vi "S-TI-S JJ Simulation.vi"() -> ()   [LabVIEW 2023]
doc: "1. before run, set the paramaters on the left of the screen.\n2. flux (magnetic field) is in unit of flux quanta.\n3. Phaserange is in the unit of Pi, the CPR will be build up according to phase range of [-Phaserange/2,Phaserang/2], and such CPR will be a periodic function with Phaserange as period. Enter integer number of multiple times of 4 is preferred.\n4. Use the step setting tab to set resolution of the calculation, you can set how many points is used to define the width of the Josephson junction, how many points to represent the Phaserange\n5. Then you can choose which type of the CPR is used.\n6. Depending on the choose of the CPR, you may want to set the strength of the MBS, \"a\" parameter, the width of the gaussian function used, and the pattern of parity of MBS. Parity pattern has to have same number of elements for positive and negative range.\nEnter the parity 1 or -1 for positive and negative phase +-Pi, +-3Pi, +-5Pi etc.. in to the two arrays.\n7. You can use the index control to read the array elements, then enter the value, you can also delete an element of array by right click, the number of array elements is not limited.\n8. You can change the x,y range, zoom, create cursor etc. to help analyse the plot. Right click to save the data into excel.\n\nEnjoy!\nGuang Yue\ngyue@illinois.edu"
uses:
  dllparameter.ctl
  remove last element_plots.vi
  remove last element_2Darray.vi
panel:
  out "Current Disorder":T1={"Step width"=0.2, "App"=0.1, "Array"=[1.0078411649904462, 1.0078411649904462, 0.9846991573254764, 0.9846991573254764, 0.9978814600222632, 0.9978814600222632, 0.9723089162683902, 0.9723089162683902, 1.011631648566163, 1.011631648566163]}
  in  "Tab Control":T2(tab)
  in  "flux start":dbl=-5.0
  in  "flux end":dbl=5.0
  in  "flux step":dbl=0.1
  in  "Geometry steps":i32=201
  in  "Phase steps":i32=201
  in  "CPR Type":T3(ring)
  in  "CPR plot points":i32=500
  in  "parity for negative phase":i32[](array[numeric])=[1, -1, -1, 1]
  in  "Strenth of MBS":dbl=0.5
  in  "parity for positive phase":i32[](array[numeric])=[1, -1, 1, 1]
  in  "Gaussian width":dbl=0.2
  in  "Plot CPR":bool
  in  "Set Disorder":bool
  out "Actual flux":dbl
  in  "Flux":dbl
  in  "Plot choice":enum32{"Icp", "Icn"}(radio)
  in  "Geometry Disorder Type":u16(ring) items=["Disorder OFF", "Disorder ON"]
  in  "Plot J vs y":bool
  out "error out":errorcluster
  in  "clear last":bool
  in  "clear tab":bool
  in  "clear All":bool
  out "Negative Phase0":dbl
  out "phaserange in Pi":i32=16
  out "Positive Phase0":dbl
  in  "Plot tab":T4(tab)
  out "Diffraction pattern plot":cluster{cluster{dbl, "icn":dbl}[]}[](graph)
  out "Phase0 vs Flux":cluster{cluster{dbl, "icn":dbl}[]}[](graph)
  out "J vs y":cluster{cluster{dbl, "icn":dbl}[]}[](graph)
  out "CPR":cluster{cluster{dbl, "icn":dbl}[]}[](graph)
  out "Disorder":dbl[][](graph)
  in  "Save":bool
  in  "hold":bool=TRUE
  out "Current Flux":dbl=5.0
  out "Remaining steps":i32
  in  "Exit":bool
  in  "Run":bool
  out "Total time s":dbl=5.020437899999706 format="%#_5g"
  in  "stop":bool
  out "Ic negative":dbl=-0.0009989221220817583
  out "Ic positive":dbl=0.000998922122081775 format="%#_5f"
  # "Go to Help menu for instructions, \nor move your mouse cursor on the \nobject for some tip."
  # "Calculate Diffraction pattern"
  # "Version 2.1"
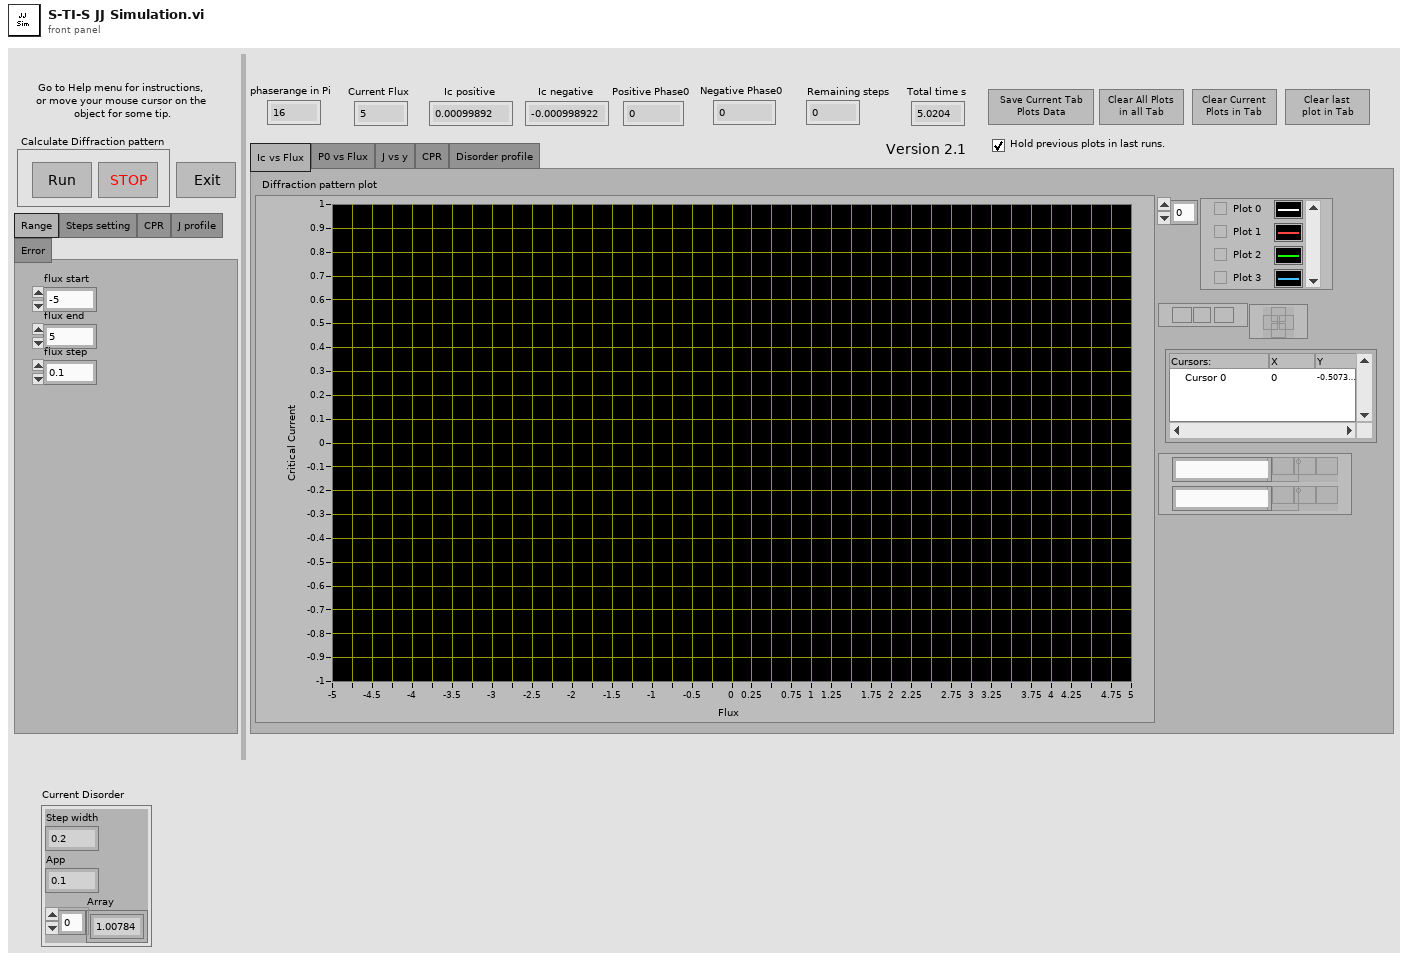
[diagram p1: front panel]
types:
  T1 = cluster{"Step width":dbl, "App":dbl, "Array":dbl[]}
  T2 = enum32{"Range", "Steps setting", "CPR", "J profile", "Error"}
  T3 = enum16{"Regular Josephson effect", "Non-local MBS", "Local MBS same parity", "Local MBS different parity"}
  T4 = enum32{"Ic vs Flux", "P0 vs Flux", "J vs y", "CPR", "Disorder profile"}
  T5 = enum8{"Enabled", "Disabled", "Disabled and Grayed Out"}
  T6 = typedef "dllparameter.ctl" = cluster{"Gaussian width":dbl, "Strenth of MBS":dbl, "Phase steps":i32, "Geometry steps":i32, "Geometry Noise Type":u16, "CPR Type":dbl, "parity for positive phase":dbl[], "parity for negative phase ":dbl[]}
  T7 = cluster{cluster{"phase":dbl, "return type":dbl}[]}
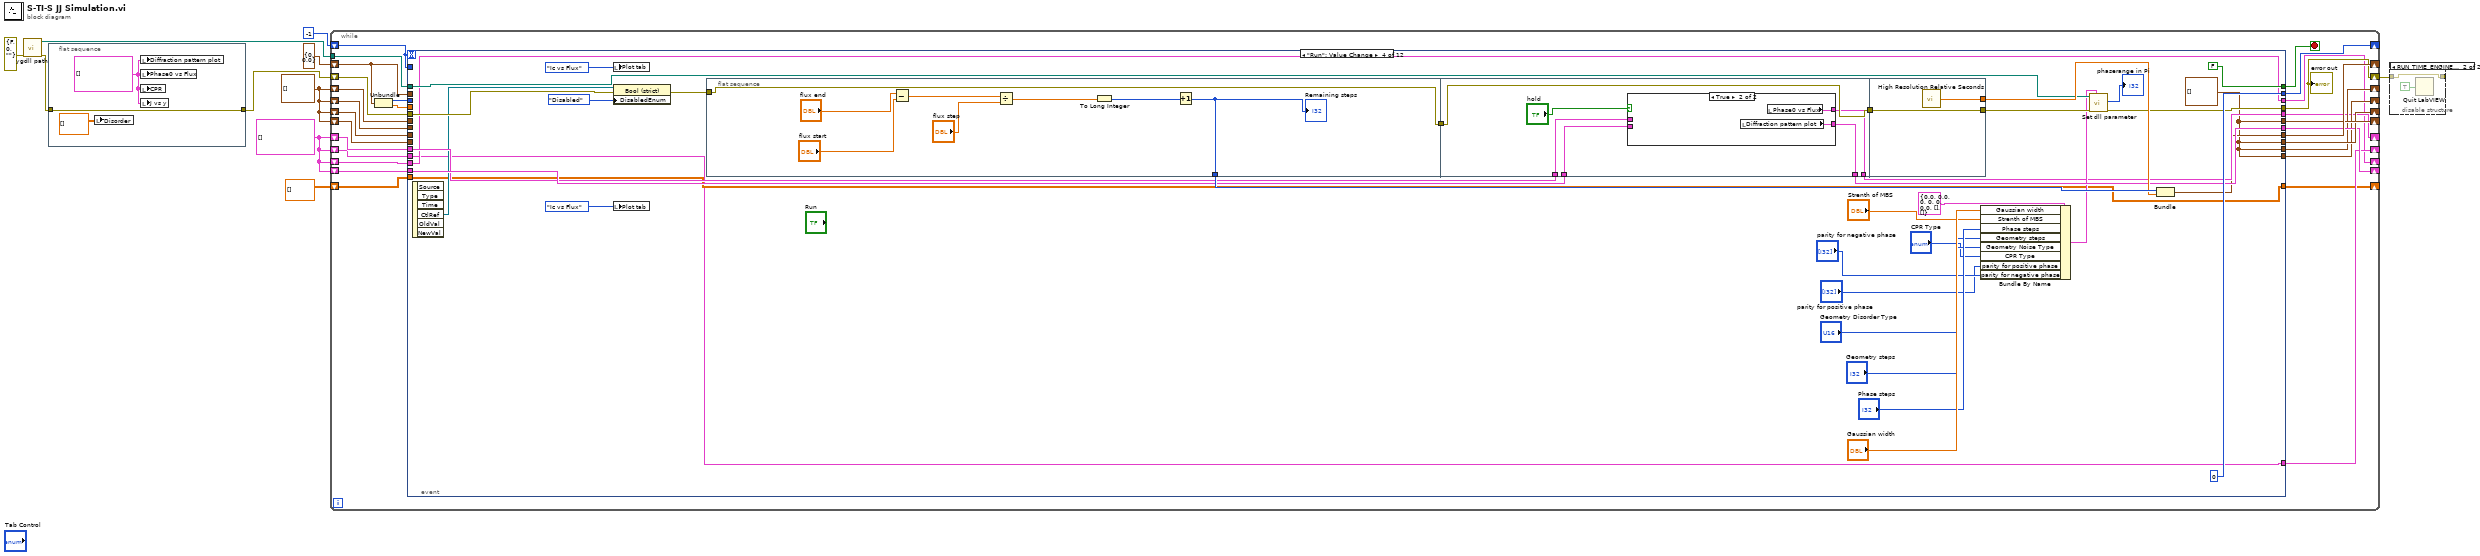
[diagram p0: block diagram]
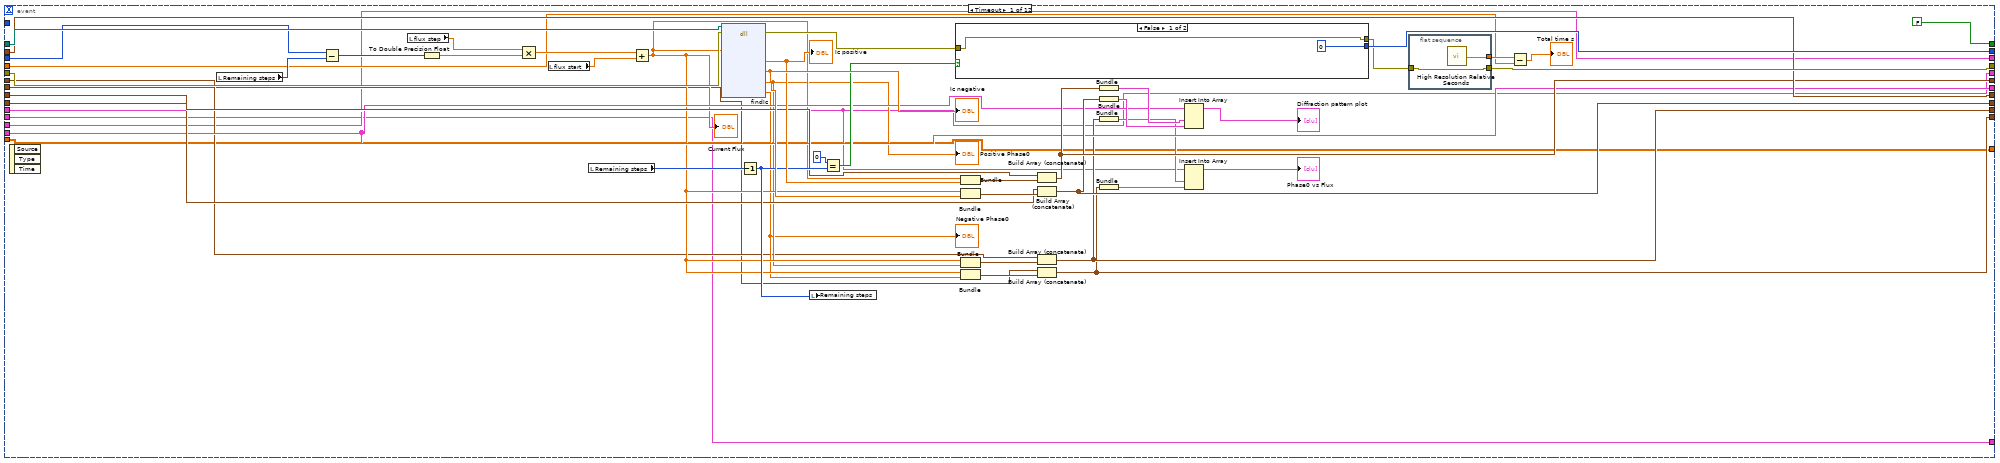
[diagram p3: hidden frame]
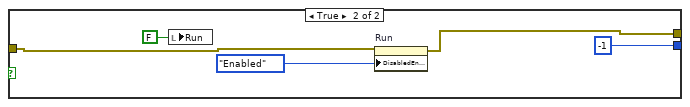
[diagram p4: hidden frame]
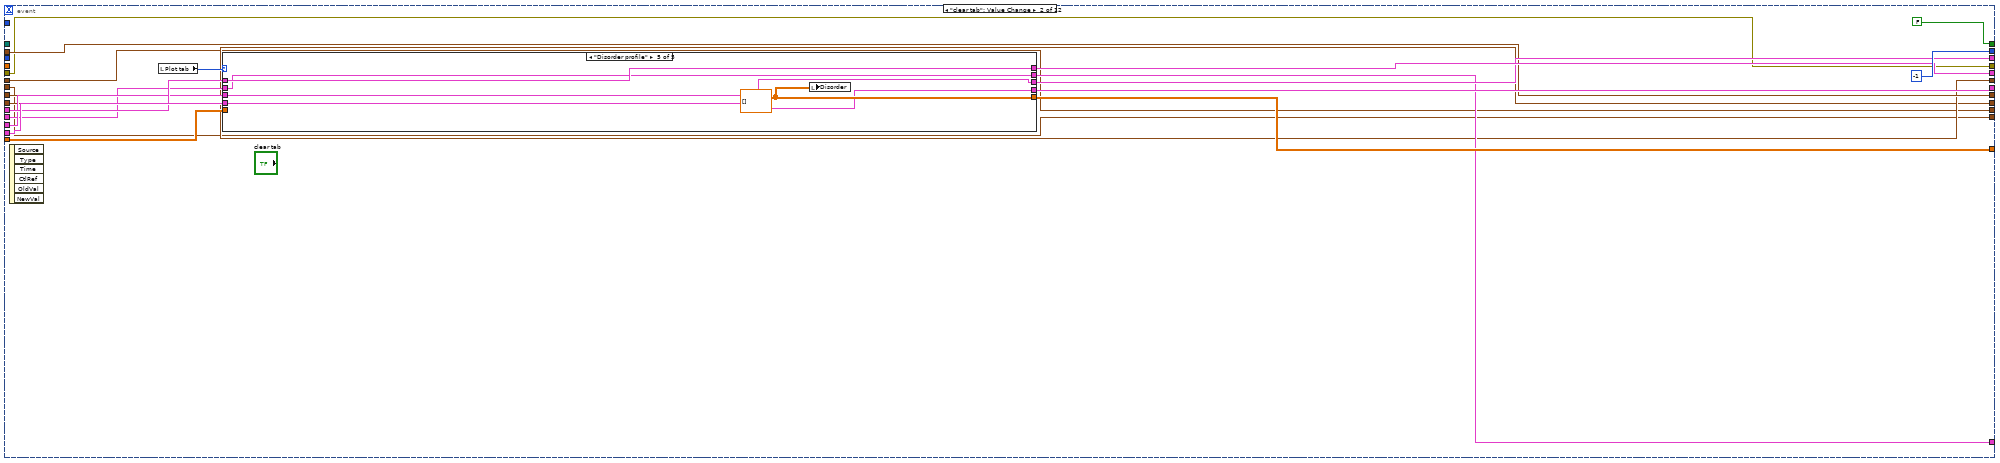
[diagram p5: hidden frame]
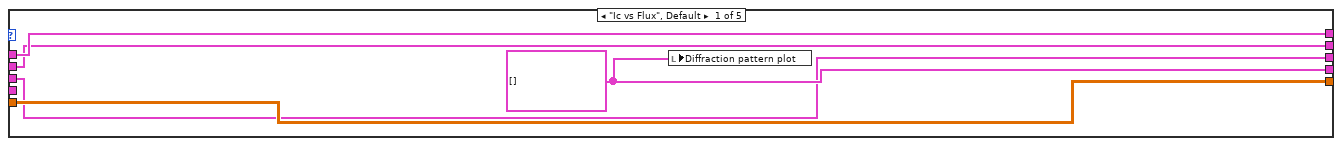
[diagram p6: hidden frame]
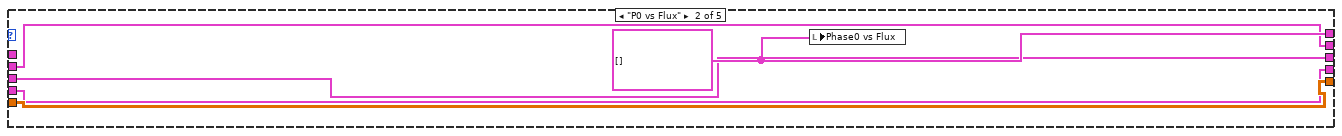
[diagram p7: hidden frame]
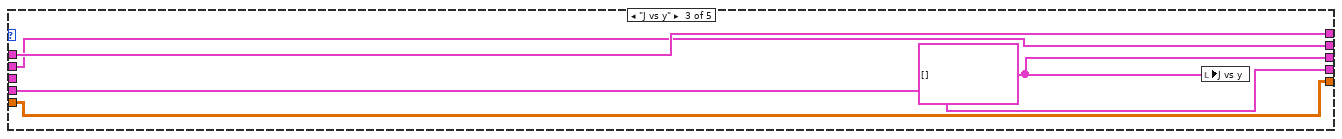
[diagram p8: hidden frame]
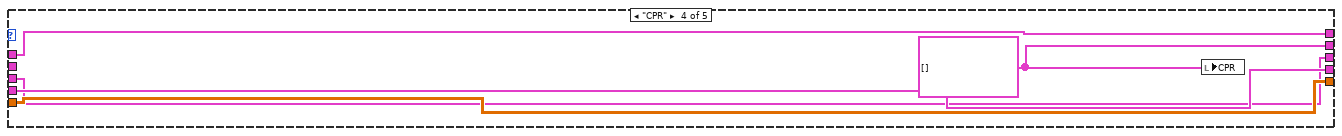
[diagram p9: hidden frame]
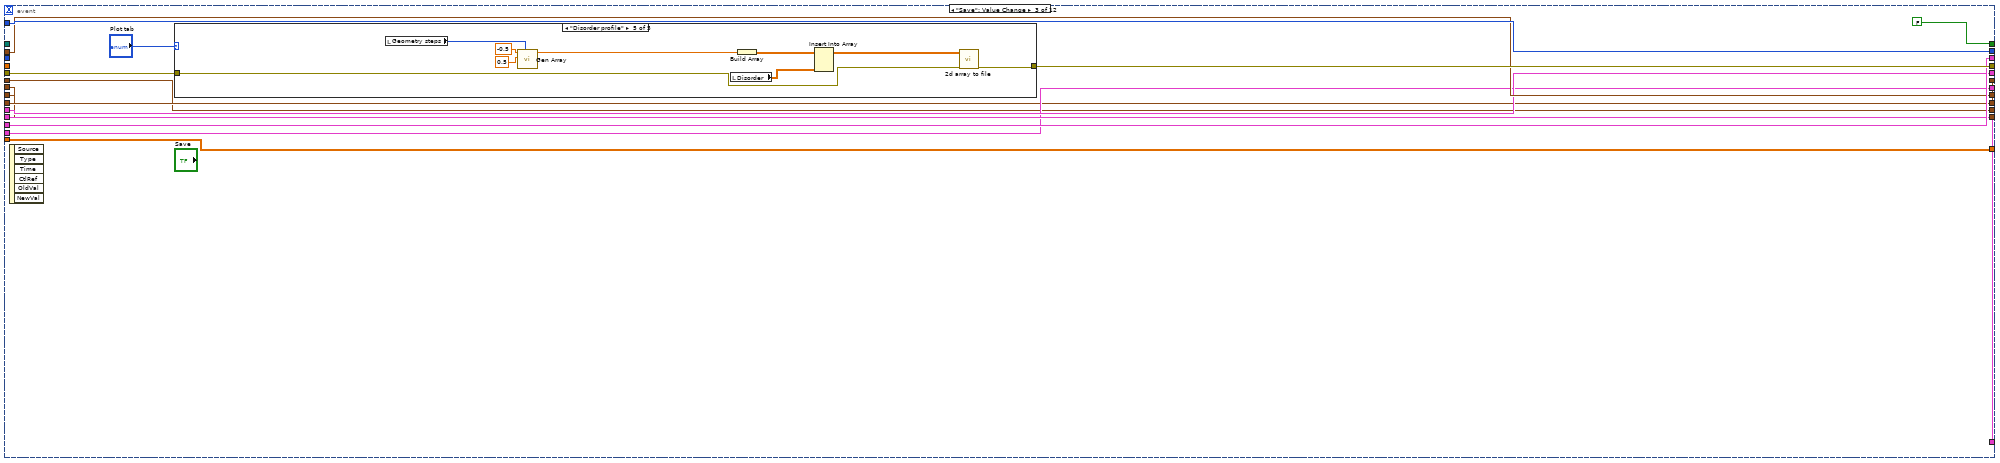
[diagram p10: hidden frame]
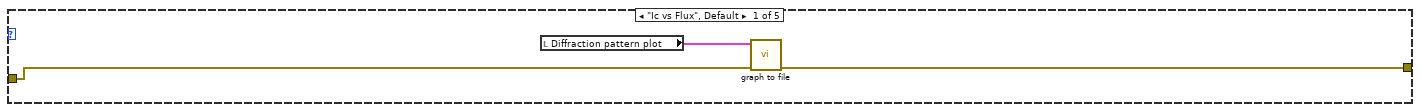
[diagram p11: hidden frame]
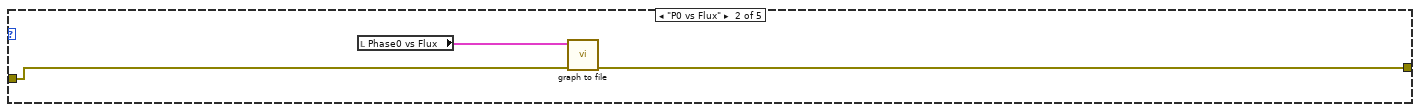
[diagram p12: hidden frame]
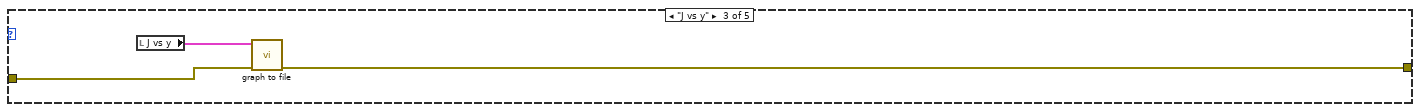
[diagram p13: hidden frame]
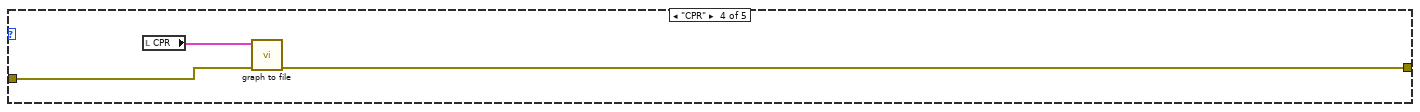
[diagram p14: hidden frame]
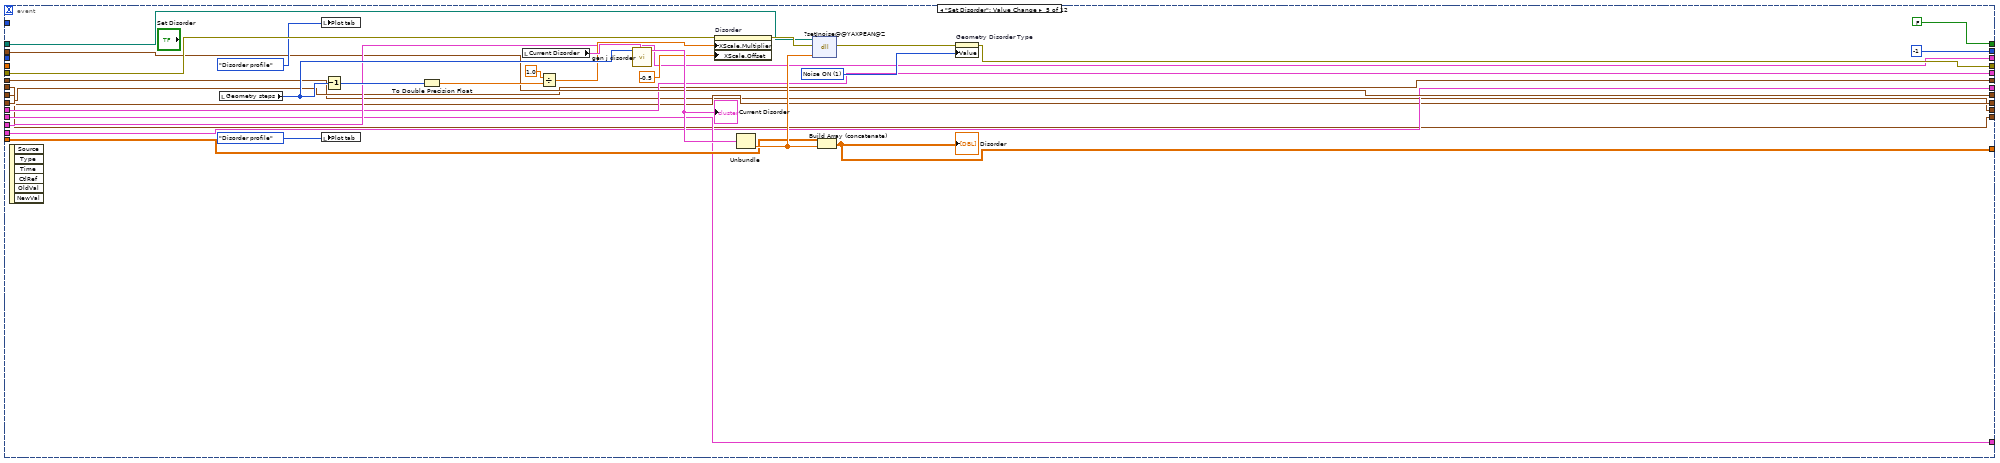
[diagram p16: hidden frame]
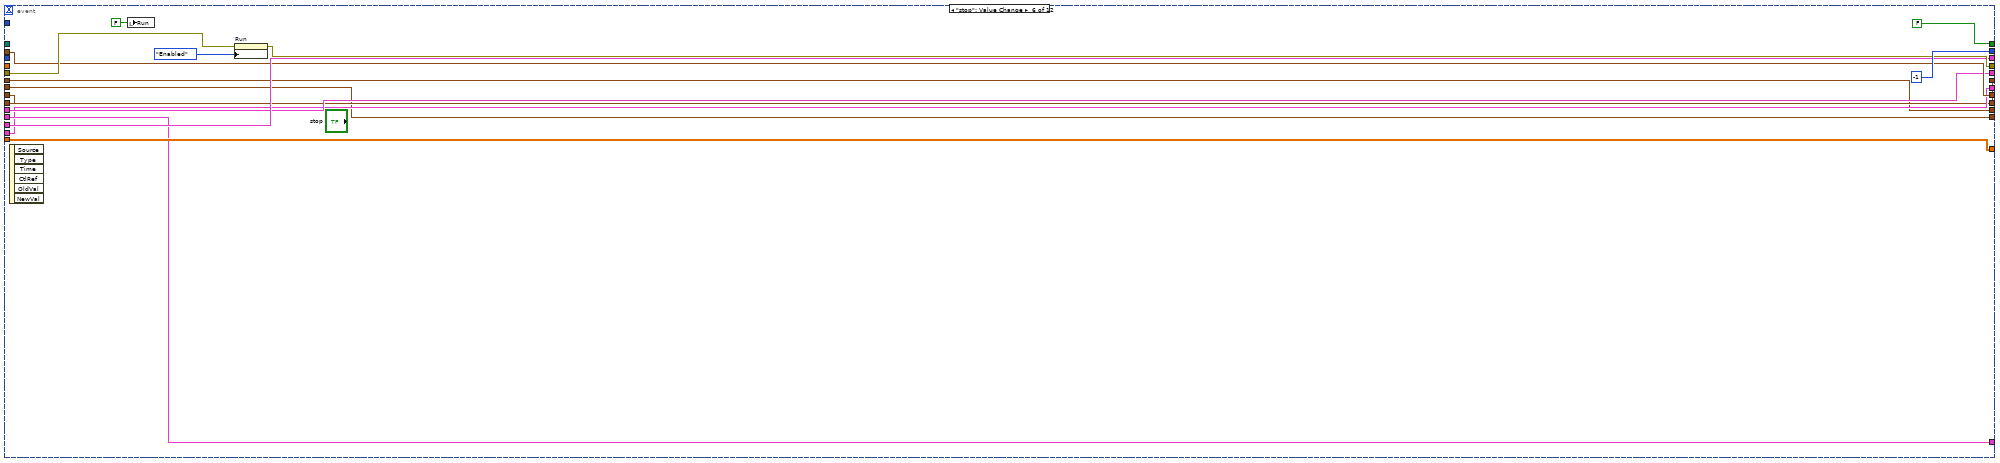
[diagram p17: hidden frame]
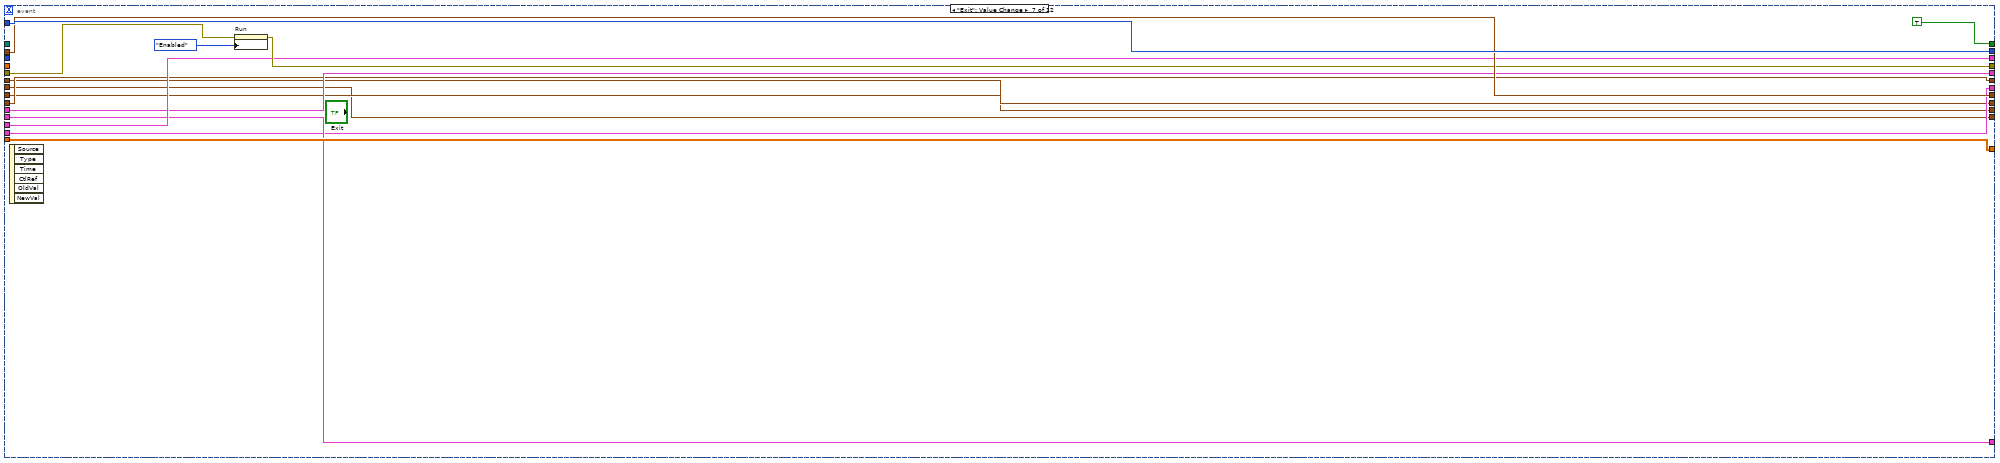
[diagram p18: hidden frame]
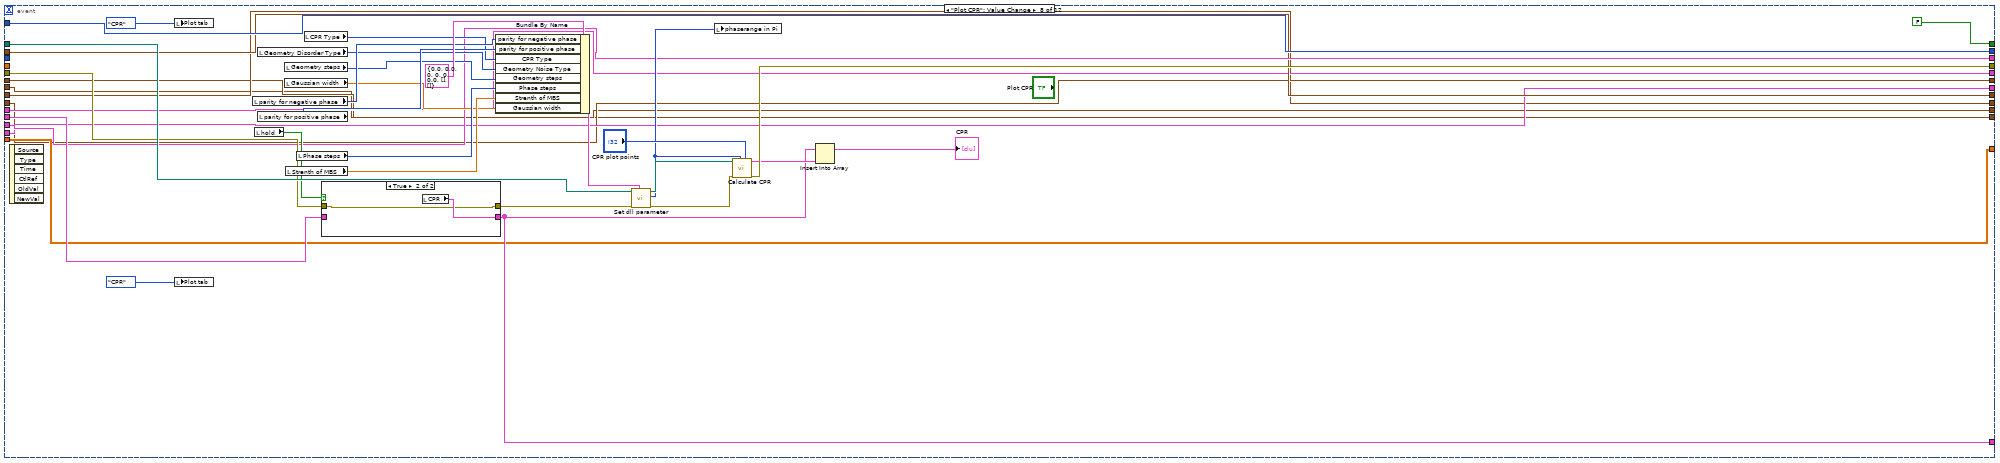
[diagram p19: hidden frame]
diagram:
  w2 = cluster{cluster{dbl, "icn":dbl}[]}[] [] ("appended array")
  w3 = cluster{dbl, "inp":dbl}[] []
  n1 = call "ygdll path.vi"("error in (no error)"=errorcluster {"status"=FALSE, "code"=0, "source"=""} ("error out")) -> ("error out"=w6:errorcluster, "appended path"=w9:path)  [unwired: 9 in]
  n2 = flat-sequence {
    tunnel: w6 -> [w13]
    tunnel: [w13] -> w5
    frame #0 {
      w12 = cluster{cluster{dbl, "icn":dbl}[]}[] [] ("appended array")
      n3 = local write "Disorder"(dbl[][] [] ("Disorder")) -> ()
      n4 = local write "Diffraction pattern plot"(w12) -> ()
      n5 = local write "Phase0 vs Flux"(w12) -> ()
      n6 = local write "CPR"(w12) -> ()
      n7 = local write "J vs y"(w12) -> ()
    }
  }
  n8 = while {
    tunnel: w9 -> [w38]
    shift-right: [w40] -> _
    shift-left: -1 -> [w33]
    shift-right: [w41] -> _
    shift-left: cluster{i32, "relative seconds":dbl} {0, "relative seconds"=0.0} ("output cluster") -> [w34]
    shift-right: [w36] -> w7
    shift-left: w5 -> [w39]
    shift-right: [w31] -> _
    shift-left: w3 -> [w32]
    shift-right: [w30] -> _
    shift-left: w3 -> [w29]
    shift-right: [w26] -> _
    shift-left: w2 -> [w27]
    shift-right: [w23] -> _
    shift-left: w3 -> [w25]
    shift-right: [w22] -> _
    shift-left: w3 -> [w24]
    shift-right: [w20] -> _
    shift-left: w2 -> [w21]
    shift-right: [w18] -> _
    shift-left: w2 -> [w19]
    shift-right: [w16] -> _
    shift-left: w2 -> [w17]
    shift-right: [w14] -> _
    shift-left: dbl[][] [] -> [w15]
    stop <- w28 stop-if-true
    n9 = Unbundle(w34) -> (w35:i32, "relative seconds"=w37:dbl)
    n10 = event shown="[3] \"Run\": Value Change" {
      selector: _ -> [_ _ _ _ _ _ _ _ _ _ _ _]
      dyn-events: _ -> [_ _ _ _ _ _ _ _ _ _ _ _]
      timeout: w33 -> [_ _ _ _ _ _ _ _ _ _ _ _]
      tunnel: [w69 w106 w152 w190 w244 w273 w295 w303 w342 w352 w403 w440] -> w41
      tunnel: [w71 -1 w158 0 -1 -1 w296 w330 -1 -1 -1 w447] -> w40
      tunnel: w39 -> [w84 w105 w156 w211 w255 w280 w293 w313 w341 w351 w411 w446]
      tunnel: w38 -> [w83 _ _ w203 w236 _ _ w328 _ _ w424 _]
      tunnel: w37 -> [w58 _ _ _ _ _ _ _ _ _ _ _]
      tunnel: [w82 w105 w155 w201 w263 w278 w291 w331 w341 w351 w414 w445] -> w36
      tunnel: w35 -> [w81 _ _ _ _ _ _ _ _ _ _ _]
      tunnel: w34 -> [w69 w106 w152 _ w244 w273 w295 w303 w342 w352 w403 w440]
      tunnel: w33 -> [_ _ w158 _ _ _ w296 w330 _ _ _ w447]
      tunnel: w32 -> [w66 w104 w148 _ w240 w269 w285 w300 w340 w350 w399 w436]
      tunnel: [w67 w104 w148 w189 w240 w269 w285 w300 w340 w350 w399 w436] -> w31
      tunnel: [w65 w103 w147 w189 w239 w268 w284 w299 w339 w349 w398 w435] -> w30
      tunnel: w29 -> [w64 w103 w147 _ w239 w268 w284 w299 w339 w349 w398 w435]
      tunnel: [FALSE FALSE FALSE FALSE FALSE FALSE TRUE FALSE FALSE FALSE FALSE FALSE] -> w28
      tunnel: w27 -> [w59 w114 w149 w207 w241 w270 w286 w301 _ w361 w400 w437]
      tunnel: [w59 w115 w149 w208 w241 w270 w286 w301 w344 w355 w400 w437] -> w26
      tunnel: w25 -> [w50 w102 w146 _ w238 w267 w283 w298 w338 w348 w397 w434]
      tunnel: w24 -> [w49 w101 w145 _ w237 w266 w282 w297 w337 w347 w396 w433]
      tunnel: [w48 w102 w146 w189 w238 w267 w283 w298 w338 w348 w397 w434] -> w23
      tunnel: [w47 w101 w145 w189 w237 w266 w282 w297 w337 w347 w396 w433] -> w22
      tunnel: w21 -> [w45 w112 w150 w197 w242 w271 w287 w302 _ w362 w401 w438]
      tunnel: [w45 w113 w150 w198 w242 w271 w287 w302 w344 w357 w401 w438] -> w20
      tunnel: w19 -> [w42 w108 w151 w191 w243 w272 w288 w311 _ w363 w402 w439]
      tunnel: [w42 w109 w151 w191 w243 w272 w288 w309 w344 w354 w402 w439] -> w18
      tunnel: w17 -> [w43 w110 w153 w192 w246 w274 w289 w305 _ w360 w409 w442]
      tunnel: [w43 w111 w153 w192 w246 w274 w289 w305 w344 w358 w408 w442] -> w16
      tunnel: w15 -> [w44 w116 w154 w193 w257 w275 w290 w306 _ w356 w405 w443]
      tunnel: [w44 w117 w154 w193 w256 w275 w290 w306 w345 w359 w405 w443] -> w14
      event Timeout {
        n11 = event-data() -> ()  [unwired: 1 in, 3 out]
        n12 = local read "Remaining steps"() -> (w80:i32)
        n13 = Subtract(x=w81, y=w80) -> (x-y=w78:i32)
        n14 = local read "flux step"() -> (w79:dbl)
        n15 = To Double Precision Float(number=w78) -> (double precision float=w87:dbl)
        n16 = Multiply(x=w79, y=w87) -> (x*y=w88:dbl)
        n17 = local read "flux start"() -> (w77:dbl)
        n18 = local read "Remaining steps"() -> (w75:i32)
        n19 = Add(x=w88, y=w77) -> (x+y=w53:dbl)
        "Current Flux" <- w53
        n20 = dll-call lib="C:/Users/yg/Box/Guang Yue uiuc research box folder/computation/S-TI-S jj simulation c/Release/ygDLL.dll" fn="findIc"(path in=w83, error in=w84, "flux"=w53) -> (error out=w76:errorcluster, "inp"=w89:dbl, "icn"=w90:dbl, "pp0"=w52:dbl, "pn0"=w51:dbl)  [unwired: 7 in, 1 out]
        "Ic positive" <- w89
        "Ic negative" <- w90
        "Positive Phase0" <- w52
        "Negative Phase0" <- w51
        n21 = Decrement(x=w75) -> (x-1=w73:i32)
        n22 = local write "Remaining steps"(w73) -> ()
        n23 = Equal?(x=0, y=w73) -> (x = y?=w72:bool)
        n24 = case shown="False" w72 {
          tunnel: w76 -> [w92 w97]
          tunnel: [0 -1] -> w71
          tunnel: [w92 w96] -> w70
          frame False {
          }
          frame True {
            n25 = local write "Run"(FALSE ("Run")) -> ()
            n26 = property on="Run" class="Bool (strict)"(error in=w97, "DisabledEnum"=T5."Enabled" ("Disabled")) -> (error out=w96:errorcluster)  [unwired: 1 in, 1 out]
          }
        }
        n27 = Bundle(w53, "inp"=w89) -> (w68:cluster{dbl, "inp":dbl})  [unwired: 1 in]
        n28 = Bundle(w53, "icn"=w90) -> (w91:cluster{dbl, "icn":dbl})  [unwired: 1 in]
        n29 = Bundle(w53, "pp0"=w52) -> (w56:cluster{dbl, "pp0":dbl})  [unwired: 1 in]
        n30 = Bundle(w53, "pn0"=w51) -> (w57:cluster{dbl, "pn0":dbl})  [unwired: 1 in]
        n31 = Build Array (concatenate)(w66, w68) -> (w67:cluster{dbl, "inp":dbl}[])
        n32 = Build Array (concatenate)(w64, w91) -> (w65:cluster{dbl, "icn":dbl}[])
        n33 = Build Array (concatenate)(w50, w56) -> (w48:cluster{dbl, "pp0":dbl}[])
        n34 = Build Array (concatenate)(w49, w57) -> (w47:cluster{dbl, "pn0":dbl}[])
        n35 = Bundle(w67) -> (w62:cluster{cluster{dbl, "inp":dbl}[]})  [unwired: 1 in]
        n36 = Bundle(w65) -> (w61:cluster{cluster{dbl, "icn":dbl}[]})  [unwired: 1 in]
        n37 = Bundle(w48) -> (w55:cluster{cluster{dbl, "pp0":dbl}[]})  [unwired: 1 in]
        n38 = Bundle(w47) -> (w54:cluster{cluster{dbl, "pn0":dbl}[]})  [unwired: 1 in]
        n39 = Insert Into Array(array=w59, new element #1=w62, new element #2=w61) -> (→"Diffraction pattern plot":cluster{cluster{dbl, "icn":dbl}[]}[])  [unwired: 1 in]
        n40 = Insert Into Array(array=w45, new element #1=w55, new element #2=w54) -> (→"Phase0 vs Flux":cluster{cluster{dbl, "icn":dbl}[]}[])  [unwired: 1 in]
        n41 = flat-sequence {
          tunnel: w70 -> [w100]
          tunnel: [w100] -> w82
          tunnel: [w99] -> w86
          frame #0 {
            n42 = call <vilib>:"High Resolution Relative Seconds.vi"() -> ("relative seconds"=w99:dbl)
          }
        }
        n43 = Subtract(x=w86, y=w58) -> (x-y=→"Total time s":dbl)
      }
      event "clear tab": Value Change {
        n44 = event-data() -> ()  [unwired: 1 in, 6 out]
        n45 = local read "Plot tab"() -> (w118:T4)
        n46 = case shown="\"Disorder profile\"" w118 {
          tunnel: [w124 w129 w134 w139 w144] -> w117
          tunnel: w116 -> [w124 w129 w134 w139 _]
          tunnel: [w123 w128 w133 w138 w143] -> w115
          tunnel: w114 -> [_ w128 w133 w138 w143]
          tunnel: [w122 w127 w132 w137 w142] -> w113
          tunnel: w112 -> [w122 _ w132 w137 w142]
          tunnel: [w121 w126 w131 w136 w141] -> w111
          tunnel: w110 -> [w121 w126 _ w136 w141]
          tunnel: [w120 w125 w130 w135 w140] -> w109
          tunnel: w108 -> [w120 w125 w130 _ w140]
          frame "Ic vs Flux", Default {
            w123 = cluster{cluster{dbl, "icn":dbl}[]}[] [] ("Diffraction pattern plot")
            n47 = local write "Diffraction pattern plot"(w123) -> ()
          }
          frame "P0 vs Flux" {
            w127 = cluster{cluster{dbl, "icn":dbl}[]}[] [] ("Phase0 vs Flux")
            n48 = local write "Phase0 vs Flux"(w127) -> ()
          }
          frame "J vs y" {
            w131 = cluster{cluster{dbl, "icn":dbl}[]}[] [] ("J vs y")
            n49 = local write "J vs y"(w131) -> ()
          }
          frame "CPR" {
            w135 = cluster{cluster{dbl, "icn":dbl}[]}[] [] ("CPR")
            n50 = local write "CPR"(w135) -> ()
          }
          frame "Disorder profile" {
            w144 = dbl[][] [] ("Disorder")
            n51 = local write "Disorder"(w144) -> ()
          }
        }
      }
      event "Save": Value Change {
        n52 = event-data() -> ()  [unwired: 1 in, 6 out]
        n53 = case shown="\"Disorder profile\"" "Plot tab" {
          tunnel: w156 -> [w162 w165 w167 w171 w180]
          tunnel: [w160 w163 w166 w170 w179] -> w155
          frame "Ic vs Flux", Default {
            n54 = local read "Diffraction pattern plot"() -> (w161:cluster{cluster{dbl, "icn":dbl}[]}[])
            n55 = call "graph to file.vi"("error in (no error)"=w162, "Input array"=w161) -> ("error out"=w160:errorcluster)  [unwired: 9 in]
          }
          frame "P0 vs Flux" {
            n56 = local read "Phase0 vs Flux"() -> (w164:cluster{cluster{dbl, "icn":dbl}[]}[])
            n57 = call "graph to file.vi"("error in (no error)"=w165, "Input array"=w164) -> ("error out"=w163:errorcluster)  [unwired: 9 in]
          }
          frame "J vs y" {
            n58 = local read "J vs y"() -> (w168:cluster{cluster{dbl, "icn":dbl}[]}[])
            n59 = call "graph to file.vi"("error in (no error)"=w167, "Input array"=w168) -> ("error out"=w166:errorcluster)  [unwired: 9 in]
          }
          frame "CPR" {
            n60 = local read "CPR"() -> (w169:cluster{cluster{dbl, "icn":dbl}[]}[])
            n61 = call "graph to file.vi"("error in (no error)"=w171, "Input array"=w169) -> ("error out"=w170:errorcluster)  [unwired: 9 in]
          }
          frame "Disorder profile" {
            n62 = local read "Geometry steps"() -> (w176:i32)
            n63 = call "Gen Array.vi"("Steps"=w176, "End"=0.5, "Start"=-0.5) -> ("Array"=w175:dbl[])  [unwired: 8 in]
            n64 = local read "Disorder"() -> (w173:dbl[][])
            n65 = Build Array(w175) -> (w174:dbl[][])
            n66 = Insert Into Array(array=w174, new element=w173) -> (w172:dbl[][])  [unwired: 2 in]
            n67 = call "2d array to file.vi"("error in (no error)"=w180, "Input"=w172) -> ("error out"=w179:errorcluster)  [unwired: 9 in]
          }
        }
      }
      event "Run": Value Change {
        w189 = cluster{dbl, "inp":dbl}[] []
        n68 = event-data() -> ("CtlRef"=w196:refnum<vi>)  [unwired: 1 in, 5 out]
        n69 = local write "Plot tab"(T4."Ic vs Flux" ("Plot tab")) -> ()
        n70 = property class="Bool (strict)"(reference=w196, error in=w211, "DisabledEnum"=T5."Disabled" ("Disabled")) -> (error out=w206:errorcluster)  [unwired: 1 out]
        n71 = local write "Plot tab"(T4."Ic vs Flux" ("Plot tab")) -> ()
        n72 = flat-sequence {
          tunnel: w206 -> [w217]
          tunnel: [w216] -> w214
          tunnel: [w217] -> w205
          tunnel: w205 -> [w229]
          tunnel: [w229] -> w209
          tunnel: [w227] -> w208
          tunnel: w207 -> [w226]
          tunnel: [w225] -> w198
          tunnel: w197 -> [w224]
          tunnel: [w235] -> w204
          tunnel: w209 -> [w235]
          tunnel: [w234] -> w213
          frame #0 {
            n73 = Subtract(x="flux end", y="flux start") -> (x-y=w222:dbl)
            n74 = Divide(x=w222, y="flux step") -> (x/y=w221:dbl)
            n75 = To Long Integer(number=w221) -> (32bit integer=w220:i32)
            n76 = Increment(x=w220) -> (x+1=w216:i32)
            "Remaining steps" <- w216
          }
          frame #1 {
            n77 = case shown="True" "hold" {
              tunnel: [w231 w233] -> w227
              tunnel: w226 -> [w231 _]
              tunnel: [w230 w232] -> w225
              tunnel: w224 -> [w230 _]
              frame False {
              }
              frame True {
                n78 = local read "Diffraction pattern plot"() -> (w233:cluster{cluster{dbl, "icn":dbl}[]}[])
                n79 = local read "Phase0 vs Flux"() -> (w232:cluster{cluster{dbl, "icn":dbl}[]}[])
              }
            }
          }
          frame #2 {
            n80 = call <vilib>:"High Resolution Relative Seconds.vi"() -> ("relative seconds"=w234:dbl)
          }
        }
        n81 = Bundle By Name(cluster=T6 {"Gaussian width"=0.0, "Strenth of MBS"=0.0, "Phase steps"=0, "Geometry steps"=0, "Geometry Noise Type"=0, "CPR Type"=0.0, "parity for positive phase"=[], "parity for negative phase "=[]} ("output cluster"), "Gaussian width"="Gaussian width", "Strenth of MBS"="Strenth of MBS", "Phase steps"="Phase steps", "Geometry steps"="Geometry steps", "Geometry Noise Type"="Geometry Disorder Type", "CPR Type"="CPR Type", "parity for positive phase"="parity for positive phase", "parity for negative phase"="parity for negative phase") -> (w202:T6)
        n82 = call "Set dll parameter.vi"("Parameter Cluster"=w202, "error in (no error)"=w204, "path in"=w203) -> ("error out"=w201:errorcluster, "phaserange in Pi"=→"phaserange in Pi":i32)  [unwired: 6 in, 1 out]
        n83 = Bundle(w214, "relative seconds"=w213) -> (w190:cluster{i32, "relative seconds":dbl})  [unwired: 1 in]
      }
      event "Set Disorder": Value Change {
        w262 = u16 1 items=["Noise OFF", "Noise ON"] ("Geometry Noise Type")
        n84 = event-data() -> ()  [unwired: 1 in, 6 out]
        n85 = local read "Geometry steps"() -> (w251:i32)
        n86 = local write "Plot tab"(T4."Disorder profile" ("Plot tab")) -> ()
        n87 = local write "Plot tab"(T4."Disorder profile" ("Plot tab")) -> ()
        n88 = Decrement(x=w251) -> (x-1=w250:i32)
        n89 = To Double Precision Float(number=w250) -> (double precision float=w249:dbl)
        n90 = local read "Current Disorder"() -> (w260:T1)
        n91 = Divide(x=1.0, y=w249) -> (x/y=w248:dbl)
        n92 = call "gen j disorder.vi"("Input"=w260, "Points"=w251) -> ("Output"=w261:T1)  [unwired: 9 in]
        "Current Disorder" <- w261
        n93 = property on="Disorder" class="WFGraph (strict)"(error in=w255, "XScale.Multiplier"=w248, "XScale.Offset"=-0.5 ("X Scale.Offset and Multiplier:Offset")) -> (error out=w254:errorcluster)  [unwired: 1 in, 1 out]
        n94 = Unbundle(w261) -> ("Array"=w258:dbl[])  [unwired: 2 out]
        n95 = dll-call lib="C:/Users/yg/Desktop/S-TI-S-simulation-C-code/x64/Release/ygDLL.dll" fn="?setJnoise@@YAXPEAN@Z"(path in=w236, error in=w254, "arg1"=w258) -> (error out=w264:errorcluster)  [unwired: 3 in, 1 out]
        n96 = Build Array (concatenate)(w257, w258) -> (w256:dbl[][])
        "Disorder" <- w256
        n97 = property on="Geometry Disorder Type" class="Ring (strict)"(error in=w264, "Value"=w262) -> (error out=w263:errorcluster)  [unwired: 1 in, 1 out]
      }
      event "stop": Value Change {
        n98 = event-data() -> ()  [unwired: 1 in, 6 out]
        n99 = local write "Run"(FALSE ("Run")) -> ()
        n100 = property on="Run" class="Bool (strict)"(error in=w280, "DisabledEnum"=T5."Enabled" ("Disabled")) -> (error out=w278:errorcluster)  [unwired: 1 in, 1 out]
      }
      event "Exit": Value Change {
        n101 = event-data() -> ()  [unwired: 1 in, 6 out]
        n102 = property on="Run" class="Bool (strict)"(error in=w293, "DisabledEnum"=T5."Enabled" ("Disabled")) -> (error out=w291:errorcluster)  [unwired: 1 in, 1 out]
      }
      event "Plot CPR": Value Change {
        n103 = event-data() -> ()  [unwired: 1 in, 6 out]
        n104 = local write "Plot tab"(T4."CPR" ("Plot tab")) -> ()
        n105 = local write "Plot tab"(T4."CPR" ("Plot tab")) -> ()
        n106 = local read "parity for negative phase"() -> (w324:i32[])
        n107 = local read "hold"() -> (w314:bool)
        n108 = local read "Geometry Disorder Type"() -> (w321:u16)
        n109 = local read "parity for positive phase"() -> (w323:i32[])
        n110 = local read "Geometry steps"() -> (w320:i32)
        n111 = local read "Gaussian width"() -> (w317:dbl)
        n112 = local read "Strenth of MBS"() -> (w318:dbl)
        n113 = local read "Phase steps"() -> (w319:i32)
        n114 = local read "CPR Type"() -> (w322:T3)
        n115 = case shown="True" w314 {
          tunnel: [w334 w335] -> w312
          tunnel: w313 -> [w334 w335]
          tunnel: [w333 w336] -> w309
          tunnel: w311 -> [w333 _]
          frame False {
          }
          frame True {
            n116 = local read "CPR"() -> (w336:cluster{cluster{dbl, "icn":dbl}[]}[])
          }
        }
        n117 = Bundle By Name(cluster=T6 {"Gaussian width"=0.0, "Strenth of MBS"=0.0, "Phase steps"=0, "Geometry steps"=0, "Geometry Noise Type"=0, "CPR Type"=0.0, "parity for positive phase"=[], "parity for negative phase "=[]} ("output cluster"), "parity for negative phase"=w324, "parity for positive phase"=w323, "CPR Type"=w322, "Geometry Noise Type"=w321, "Geometry steps"=w320, "Phase steps"=w319, "Strenth of MBS"=w318, "Gaussian width"=w317) -> (w325:T6)
        n118 = call "Set dll parameter.vi"("Parameter Cluster"=w325, "error in (no error)"=w312, "path in"=w328) -> ("error out"=w329:errorcluster, "phaserange in Pi"=w316:i32, "path out"=w327:path)  [unwired: 6 in]
        n119 = local write "phaserange in Pi"(w316) -> ()
        n120 = call "Calculate CPR.vi"("steps"="CPR plot points", "phase range"=w316, "error in (no error)"=w329, "path in"=w327) -> ("error out"=w331:errorcluster, "output Plot"=w315:T7)  [unwired: 6 in]
        n121 = Insert Into Array(array=w309, new element=w315) -> (→"CPR":cluster{cluster{dbl, "icn":dbl}[]}[])  [unwired: 1 in]
      }
      event "clear All": Value Change {
        w345 = dbl[][] []
        w344 = cluster{cluster{dbl, "icn":dbl}[]}[] [] ("CPR")
        n122 = event-data() -> ()  [unwired: 1 in, 6 out]
        n123 = local write "J vs y"(w344) -> ()
        n124 = local write "CPR"(w344) -> ()
        n125 = local write "Phase0 vs Flux"(w344) -> ()
        n126 = local write "Diffraction pattern plot"(w344) -> ()
        n127 = local write "Disorder"(w345) -> ()
      }
      event "clear last": Value Change {
        n128 = event-data() -> ()  [unwired: 1 in, 6 out]
        n129 = local read "Plot tab"() -> (w364:T4)
        n130 = case shown="\"Disorder profile\"" w364 {
          tunnel: [w371 w377 w383 w384 w391] -> w359
          tunnel: w356 -> [w371 w377 w383 _ w391]
          tunnel: [w366 w376 w382 w389 w393] -> w355
          tunnel: w361 -> [_ w376 w382 w389 w393]
          tunnel: [w370 w372 w381 w388 w390] -> w357
          tunnel: w362 -> [w370 _ w381 w388 w390]
          tunnel: [w369 w375 w378 w387 w394] -> w358
          tunnel: w360 -> [w369 w375 _ w387 _]
          tunnel: [w368 w374 w380 w386 w392] -> w354
          tunnel: w363 -> [w368 w374 w380 w386 w392]
          frame "Ic vs Flux", Default {
            n131 = local read "Diffraction pattern plot"() -> (w367:cluster{cluster{dbl, "icn":dbl}[]}[])
            n132 = call-poly "remove last plot.vi"("Input"=w367) -> ("subarray"=w366:cluster{cluster{dbl, "icn":dbl}[]}[])  [unwired: 10 in]
            n133 = local write "Diffraction pattern plot"(w366) -> ()
          }
          frame "P0 vs Flux" {
            n134 = local read "Phase0 vs Flux"() -> (w373:cluster{cluster{dbl, "icn":dbl}[]}[])
            n135 = call-poly "remove last plot.vi"("Input"=w373) -> ("subarray"=w372:cluster{cluster{dbl, "icn":dbl}[]}[])  [unwired: 10 in]
            n136 = local write "Phase0 vs Flux"(w372) -> ()
          }
          frame "CPR" {
            n137 = local read "CPR"() -> (w379:cluster{cluster{dbl, "icn":dbl}[]}[])
            n138 = call-poly "remove last plot.vi"("Input"=w379) -> ("subarray"=w378:cluster{cluster{dbl, "icn":dbl}[]}[])  [unwired: 10 in]
            n139 = local write "CPR"(w378) -> ()
          }
          frame "Disorder profile" {
            n140 = local read "Disorder"() -> (w385:dbl[][])
            n141 = call-poly "remove last plot.vi"("Input"=w385) -> ("subarray"=w384:dbl[][])  [unwired: 10 in]
            n142 = local write "Disorder"(w384) -> ()
          }
          frame "J vs y" {
            n143 = local read "J vs y"() -> (w395:cluster{cluster{dbl, "icn":dbl}[]}[])
            n144 = call-poly "remove last plot.vi"("Input"=w395) -> ("subarray"=w394:cluster{cluster{dbl, "icn":dbl}[]}[])  [unwired: 10 in]
            n145 = local write "J vs y"(w394) -> ()
          }
        }
      }
      event "Plot J vs y": Value Change {
        n146 = event-data() -> ()  [unwired: 1 in, 6 out]
        n147 = local write "Plot tab"(T4."J vs y" ("Plot tab")) -> ()
        n148 = local write "Plot tab"(T4."J vs y" ("Plot tab")) -> ()
        n149 = local read "Phase0 vs Flux"() -> (w422:cluster{cluster{dbl, "icn":dbl}[]}[])
        n150 = Array Size(array=w422) -> (size(s)=w420:i32)
        n151 = case shown="\"Icp\", Default" "Plot choice" {
          tunnel: w420 -> [w430 w432]
          tunnel: [w429 w431] -> w419
          frame "Icp", Default {
            n152 = Decrement(x=w430) -> (x-1=w428:i32)
            n153 = Decrement(x=w428) -> (x-1=w429:i32)
          }
          frame "Icn" {
            n154 = Decrement(x=w432) -> (x-1=w431:i32)
          }
        }
        n155 = Index Array(array=w422, index=w419) -> (element=w418:cluster{cluster{dbl, "icn":dbl}[]})
        n156 = local read "Geometry steps"() -> (w423:i32)
        n157 = call "getfluxpoint.vi"("flux"="Flux", "Plot"=w418) -> ("phase0"=w415:dbl, "actual flux"=w416:dbl)  [unwired: 8 in]
        "Actual flux" <- w416
        n158 = call "Plot J profile.vi"("p0"=w415, "Steps"=w423, "flux"=w416, "error in (no error)"=w411, "path in"=w424) -> ("error out"=w414:errorcluster, "plot"=w413:cluster{cluster{dbl, "return type":dbl}[]})  [unwired: 4 in, 1 out]
        n159 = Build Array (concatenate)(w409, w413) -> (w410:cluster{cluster{dbl, "return type":dbl}[]}[])
        "J vs y" <- w410
        n160 = local read "hold"() -> (w412:bool)
        n161 = case shown="False" w412 {
          tunnel: w410 -> [_ w427]
          tunnel: [w426 w427] -> w408
          tunnel: w409 -> [w426 _]
          frame False {
          }
          frame True {
          }
        }
      }
      event Menu Selection (User) {
        n162 = event-data() -> ("ItemTag"=w444:string)  [unwired: 1 in, 5 out]
        n163 = case shown="\"About_me\"" w444 {
          tunnel: w446 -> [w448 w450 w454]
          tunnel: [w448 w449 w452] -> w445
          frame Default {
          }
          frame "About_me" {
            n164 = call "About this program"("error in (no error)"=w450, "Message"="This software is developed for simulation on S-TI-S Josephson junction. Majorana Bound State, iregular current phase relation are considered. The calucation results include diffraction pattern, optimised phase0, current phase relation plot, local current distribution etc.\nChange Log: \nv1.0 basic program for diffraction pattern simulation\nv1.6 Added multi-plots feature and easy data save function.\nv 2.0 Add calculation of current phase relation, optimised phase0, plot of local current. Geometry disorder on the current density along y direction.\nV2.1 Don't have to press enter before click a button, add save disorder pattern function, switch to certain plot after run, disorder subVI will remember last setting\nGuang Yue, DVH group\ngyue@illinois.edu") -> ("error out"=w449:errorcluster)  [unwired: 8 in, 1 out]
          }
          frame "Usage Instructions" {
            n165 = call <vilib>:"Application Directory.vi"() -> ("Application Directory"=w456:path)
            n166 = Build Path(base path=w456, name or relative path="S-TI-S_JJ_Simulation Help.chm") -> (appended path=w453:path)
            n167 = call <vilib>:"Open a Document on Disk.vi"("error in (no error)"=w454, "document path"=w453) -> ("error out"=w452:errorcluster)  [unwired: 5 in]
          }
        }
      }
    }
    "error out" <- w36
  }
  n168 = disable-structure shown="RUN_TIME_ENGINE==True" {
    disable-tunnel: [w457 w458] -> _
    disable-tunnel: w7 -> [w457 w458]
    frame condition #0 (active) {
    }
    frame condition #1 {
      n169 = Quit LabVIEW(quit? (T)=TRUE) -> ()
    }
  }
